vi "Column String.vi"(8 "error in (no error)":errorcluster, 11 "SQL Statement in":refnum<class "SQL Statement.lvclass">) -> (0 "error out":errorcluster, 2 "Text":string, 3 "SQL Statement out":refnum<class "SQL Statement.lvclass">)   [LabVIEW 2011, in "SQLite.lvlib" / "SQL Statement.lvclass"]
doc: "Returns the value in the next column as a LabVIEW string. Note that this ment for use with both SQLite3 TEXT and BLOB datatypes. Numeric types will be converted into text form."
uses:
  SQL Statement.lvclass
  SQL Statement.lvclass/SQL Statement.ctl
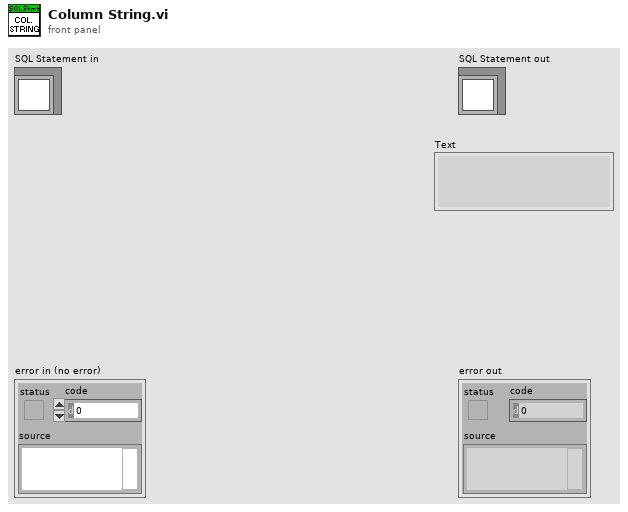
[diagram p1: front panel]
types:
  T1 = typedef "SQLite.lvlib/SQLITE Datatype.ctl" = enum32{"undefined type (0)", "SQLITE_INTEGER", "SQLITE_FLOAT", "SQLITE3_TEXT", "SQLITE_BLOB", "SQLITE_NULL", "undefined type"}
  T2 = typedef "SQLite.lvlib/SQL Statement.lvclass/Text Encoding" = enum16{"System", "UTF-8", "UTF-16"}
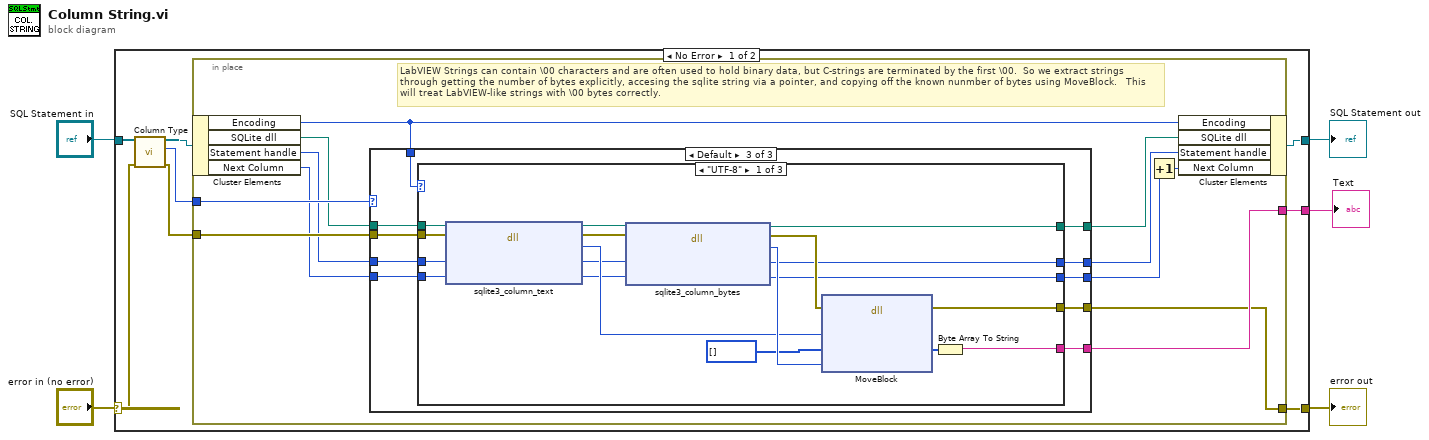
[diagram p0: block diagram]
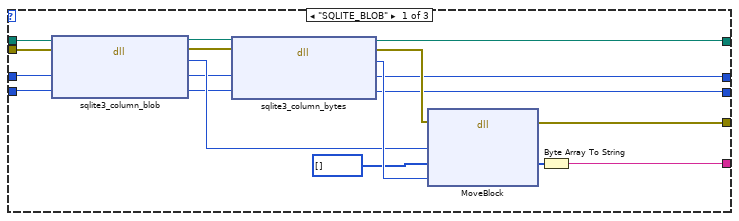
[diagram p2: hidden frame]
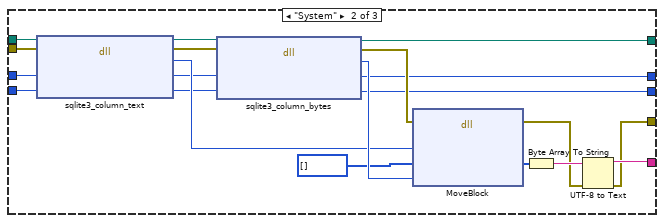
[diagram p4: hidden frame]
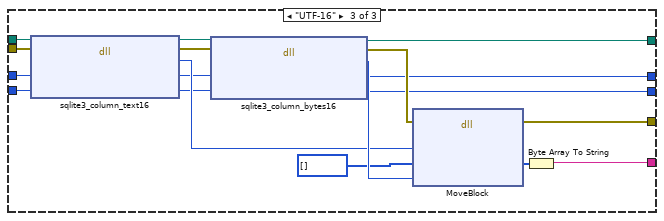
[diagram p5: hidden frame]
diagram:
  n1 = case shown="No Error" "error in (no error)" {
    selector: "error in (no error)" -> [w8 w115]
    tunnel: [w12 w115] -> w2
    tunnel: [w11 w114] -> w3
    tunnel: "SQL Statement in" -> [w10 w114]
    tunnel: [w13 _] -> w1
    frame No Error {
      n2 = call "Column Type.vi"("error in (no error)"=w8, "SQL Statement in"=w10) -> ("error out"=w7:errorcluster, "SQLite3 type"=w6:T1, "SQL Statement out"=w9:refnum<class "SQL Statement.lvclass">)  [unwired: 7 in]
      n3 = in-place {
        in-place-border: [w25] -> w13
        in-place-border: w7 -> [w17]
        in-place-border: [w24] -> w12
        in-place-border: w6 -> [w19]
        # "LabVIEW Strings can contain \\00 characters and are often used to hold binary data, but C-strings are terminated by the first \\00.  So we extract strings through getting the number of bytes explicitly, accesing the sqlite string via a pointer, and copying off the known nunmber of bytes using MoveBlock.   This will treat LabVIEW-like strings with \\00 bytes correctly."
        n4 = in-place-cluster #1(w9) -> ("Encoding"=w14:T2, "SQLite dll"=w18:path, "Statement handle"=w16:u64, "Next Column"=w15:i32)
        n5 = case shown="Default" w19 {
          tunnel: [w26 _ w57] -> w25
          tunnel: [w27 w44 w56] -> w24
          tunnel: [w30 w47 w55] -> w23
          tunnel: [w29 w46 w54] -> w22
          tunnel: [w28 w45 w53] -> w20
          tunnel: w18 -> [w31 w47 w52]
          tunnel: w17 -> [w32 w44 w51]
          tunnel: w16 -> [w34 w46 w50]
          tunnel: w15 -> [w33 w45 w49]
          tunnel: w14 -> [_ _ w48]
          frame "SQLITE_BLOB" {
            n6 = dll-call lib="C:/LabVIEW_JDP/Support/SQLite/SQL Connection/sqlite3.dll" fn="sqlite3_column_blob"(path in=w31, error in=w32, "Statement"=w34, "Column"=w33) -> (path out=w37:path, error out=w36:errorcluster, "Pointer"=w42:u64, "Statement"=w39:u64, "Column"=w38:i32)  [unwired: 1 in]
            n7 = dll-call lib="C:/LabVIEW_JDP/Support/SQLite/sqlite3.dll" fn="sqlite3_column_bytes"(path in=w37, error in=w36, "Statement"=w39, "Column"=w38) -> (path out=w30:path, error out=w35:errorcluster, "Number of Bytes"=w43:i32, "Statement"=w29:u64, "Column"=w28:i32)  [unwired: 1 in]
            n8 = dll-call lib="LabVIEW" fn="MoveBlock"(error in=w35, "Source Pointer"=w42, "Destination U8 Array"=u8[] [], "Number of Bytes"=w43) -> (error out=w27:errorcluster, "Destination U8 Array"=w41:u8[])  [unwired: 5 in, 1 out]
            n9 = Byte Array To String(unsigned byte array=w41) -> (string=w26:string)
          }
          frame "SQLITE_NULL" {
          }
          frame Default {
            n10 = case shown="\"UTF-8\"" w48 {
              tunnel: [w75 w78 w113] -> w57
              tunnel: [w74 w76 w112] -> w56
              tunnel: [w60 w82 w98] -> w55
              tunnel: [w59 w81 w97] -> w54
              tunnel: [w58 w80 w96] -> w53
              tunnel: w52 -> [w69 w91 w107]
              tunnel: w51 -> [w68 w90 w106]
              tunnel: w50 -> [w67 w89 w105]
              tunnel: w49 -> [w66 w88 w104]
              frame "UTF-8" {
                n11 = dll-call lib="C:/LabVIEW_JDP/Support/SQLite/SQL Connection/sqlite3.dll" fn="sqlite3_column_text"(path in=w69, error in=w68, "Statement"=w67, "Column"=w66) -> (path out=w63:path, error out=w62:errorcluster, "Pointer"=w72:u64, "Statement"=w65:u64, "Column"=w64:i32)  [unwired: 1 in]
                n12 = dll-call lib="C:/LabVIEW_JDP/Support/SQLite/sqlite3.dll" fn="sqlite3_column_bytes"(path in=w63, error in=w62, "Statement"=w65, "Column"=w64) -> (path out=w60:path, error out=w61:errorcluster, "Number of Bytes"=w73:i32, "Statement"=w59:u64, "Column"=w58:i32)  [unwired: 1 in]
                n13 = dll-call lib="LabVIEW" fn="MoveBlock"(error in=w61, "Source Pointer"=w72, "Destination U8 Array"=u8[] [], "Number of Bytes"=w73) -> (error out=w74:errorcluster, "Destination U8 Array"=w71:u8[])  [unwired: 5 in, 1 out]
                n14 = Byte Array To String(unsigned byte array=w71) -> (string=w75:string)
              }
              frame "System" {
                n15 = dll-call lib="C:/LabVIEW_JDP/Support/SQLite/SQL Connection/sqlite3.dll" fn="sqlite3_column_text"(path in=w91, error in=w90, "Statement"=w89, "Column"=w88) -> (path out=w85:path, error out=w84:errorcluster, "Pointer"=w94:u64, "Statement"=w87:u64, "Column"=w86:i32)  [unwired: 1 in]
                n16 = dll-call lib="C:/LabVIEW_JDP/Support/SQLite/sqlite3.dll" fn="sqlite3_column_bytes"(path in=w85, error in=w84, "Statement"=w87, "Column"=w86) -> (path out=w82:path, error out=w83:errorcluster, "Number of Bytes"=w95:i32, "Statement"=w81:u64, "Column"=w80:i32)  [unwired: 1 in]
                n17 = dll-call lib="LabVIEW" fn="MoveBlock"(error in=w83, "Source Pointer"=w94, "Destination U8 Array"=u8[] [], "Number of Bytes"=w95) -> (error out=w77:errorcluster, "Destination U8 Array"=w93:u8[])  [unwired: 5 in, 1 out]
                n18 = Byte Array To String(unsigned byte array=w93) -> (string=w79:string)
                n19 = UTF-8 to Text(8:w77, 11:w79) -> (0:w76:errorcluster, 3:w78:string)
              }
              frame "UTF-16" {
                n20 = dll-call lib="C:/LabVIEW_JDP/Support/SQLite/SQL Connection/sqlite3.dll" fn="sqlite3_column_text16"(path in=w107, error in=w106, "Statement"=w105, "Column"=w104) -> (path out=w101:path, error out=w100:errorcluster, "Pointer"=w110:u64, "Statement"=w103:u64, "Column"=w102:i32)  [unwired: 1 in]
                n21 = dll-call lib="C:/LabVIEW_JDP/Support/SQLite/SQL Connection/sqlite3.dll" fn="sqlite3_column_bytes16"(path in=w101, error in=w100, "Statement"=w103, "Column"=w102) -> (path out=w98:path, error out=w99:errorcluster, "Number of Bytes"=w111:i32, "Statement"=w97:u64, "Column"=w96:i32)  [unwired: 1 in]
                n22 = dll-call lib="LabVIEW" fn="MoveBlock"(error in=w99, "Source Pointer"=w110, "Destination U8 Array"=u8[] [], "Number of Bytes"=w111) -> (error out=w112:errorcluster, "Destination U8 Array"=w109:u8[])  [unwired: 5 in, 1 out]
                n23 = Byte Array To String(unsigned byte array=w109) -> (string=w113:string)
              }
            }
          }
        }
        n24 = Increment(x=w20) -> (x+1=w21:i32)
        n25 = in-place-cluster #1("Encoding"=w14, "SQLite dll"=w23, "Statement handle"=w22, "Next Column"=w21) -> (w11:refnum<class "SQL Statement.lvclass">)
      }
    }
    frame Error {
    }
  }
  "error out" <- w2
  "SQL Statement out" <- w3
  "Text" <- w1
